vi "WheelTest Dialog Serial with Evt.vi"(8 "error in (no error)":cluster{"状态":bool, "代码":i32, "源":string} caption="错误输入（无错误）", 11 "设置输入":T1) -> (0 "error in (no error) 2":cluster{"状态":bool, "代码":i32, "源":string} caption="错误输入（无错误）", 3 "设置输出":T1)   [LabVIEW 2012, in "Testing.lvlib"]
doc: "使用该模板构建用户界面事件处理设计模式。将模板应用于对话框及其它用户界面。用户也可创建并执行VI可按照与用户界面事件相同方式处理的用户定义事件。"
uses:
  Testing.lvlib
  Settings/Settings.ctl
  Acquisition/Hardware Configuration.ctl
  Acquisition/Signal Type.ctl
  Logging/Logging Configuration.ctl
  User_define/User_define.lvlib
  Acquisition/Acquisition.lvlib
  Logging/Logging.lvlib
  Settings/Settings.lvlib
panel:
  in  "选项卡控件":enum32{"选项卡 1", "选项卡 2"}(tab)
  in  "左后退按钮":bool
  in  "Exit":bool caption="停止"
  in  "左行走轮启停控制":bool caption="按钮1"
  in  "左行走轮速度":u8(slide) scale=0.0..100.0
  out "左行走轮速度反馈值":u16(slide) scale=0.0..100.0
  in  "左前进按钮":bool
  out "右行走轮速度反馈值":u16(slide) scale=0.0..100.0
  in  "右行走轮速度":u8(slide) scale=0.0..100.0
  in  "右行走轮启停控制":bool caption="按钮1"
  in  "右前进按钮":bool
  in  "右后退按钮":bool
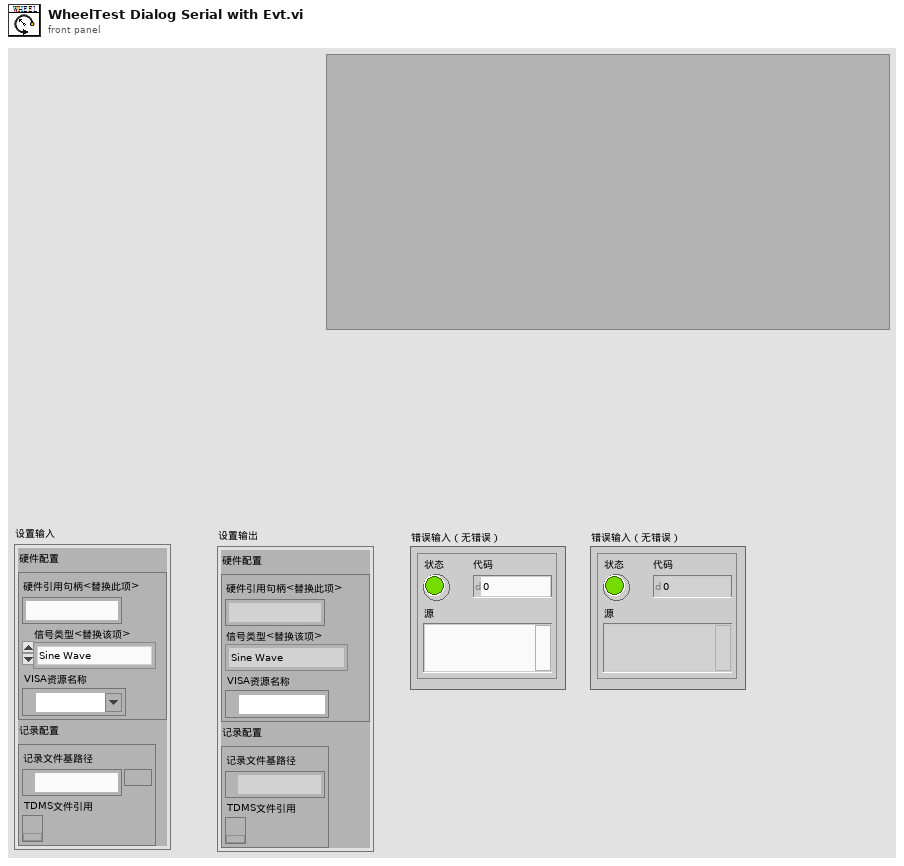
[diagram p1: front panel]
types:
  T1 = typedef "Settings.lvlib/Settings.ctl" = cluster{"硬件配置":T2, "记录配置":T4}
  T2 = typedef "Acquisition.lvlib/Hardware Configuration.ctl" = cluster{"硬件引用句柄<替换此项>":string, "信号类型<替换该项>":T3, "VISA资源名称":refnum<visa-resource-name>}
  T3 = typedef "Acquisition.lvlib/Signal Type.ctl" = enum16{"Sine Wave", "Square with Noise"}
  T4 = typedef "Logging.lvlib/Logging Configuration.ctl" = cluster{"记录文件基路径":path, "TDMS文件引用":refnum<k34>}
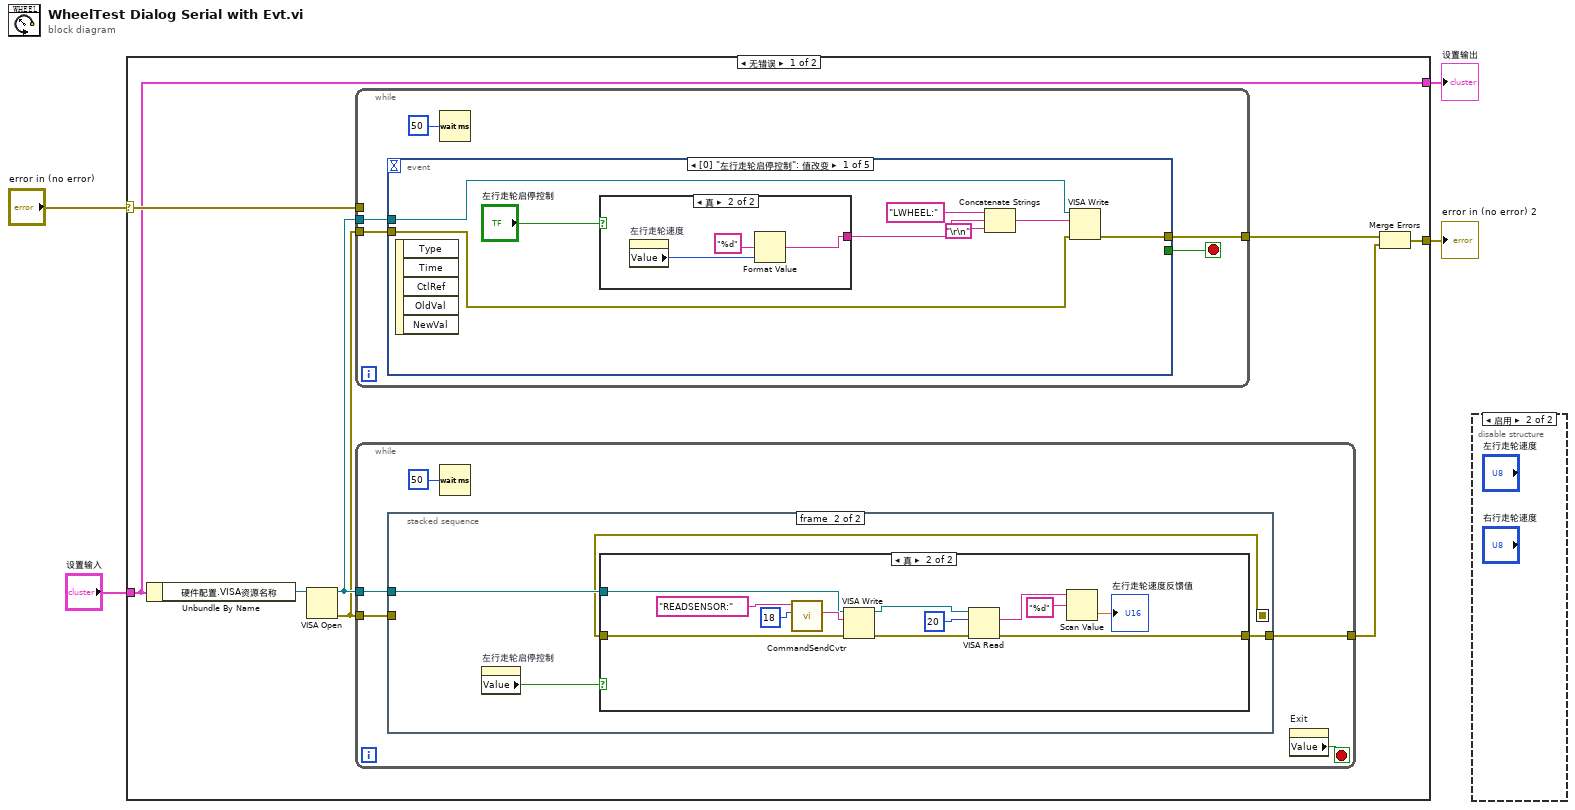
[diagram p0: block diagram]
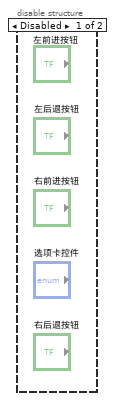
[diagram p2: hidden frame]
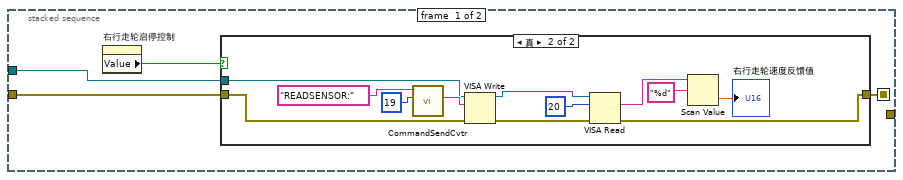
[diagram p3: hidden frame]
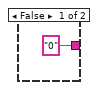
[diagram p6: hidden frame]
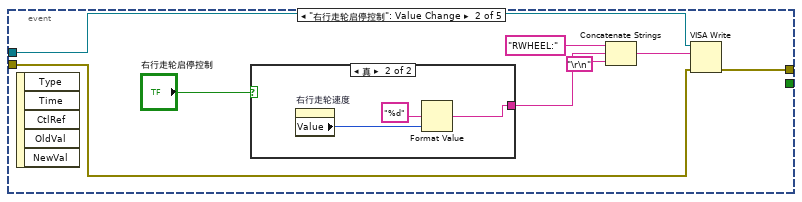
[diagram p7: hidden frame]
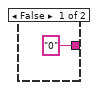
[diagram p8: hidden frame]
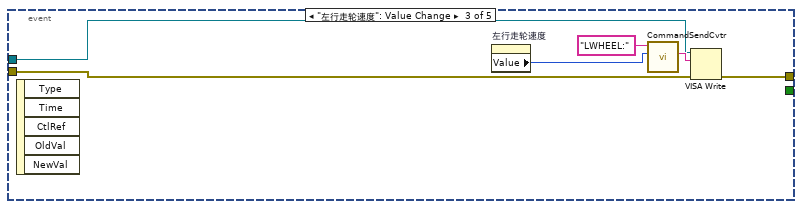
[diagram p9: hidden frame]
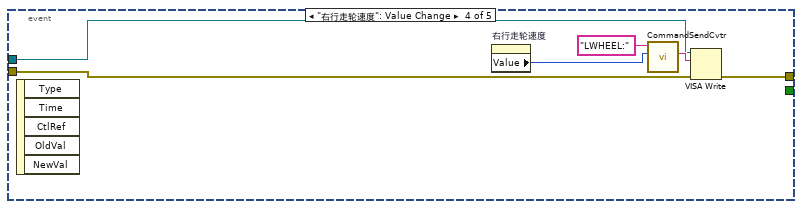
[diagram p10: hidden frame]
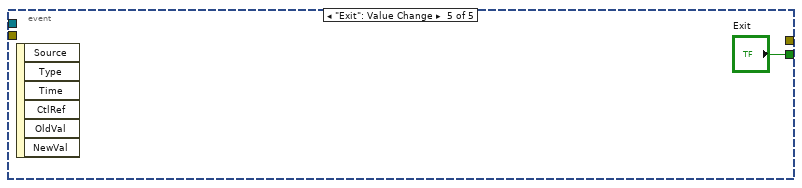
[diagram p11: hidden frame]
diagram:
  n1 = case shown="无错误" "error in (no error)" {
    selector: "error in (no error)" -> [w12 w95]
    tunnel: "设置输入" -> [w5 w94]
    tunnel: [w6 w95] -> w3
    tunnel: [w5 w94] -> w1
    frame No Error {
      n2 = Unbundle By Name(w5) -> ("硬件配置.VISA资源名称"=w11:refnum<visa-resource-name>)
      n3 = VISA Open(VISA resource name=w11) -> (VISA resource name=w10:refnum<visa-resource-name>, error out=w9:errorcluster)  [unwired: 4 in]
      n4 = while {
        tunnel: w12 -> [_]
        tunnel: w10 -> [w54]
        tunnel: w9 -> [w53]
        tunnel: [w52] -> w8
        stop <- w55 stop-if-true
        n5 = event shown="[0] \"左行走轮启停控制\": 值改变" {
          selector: _ -> [_ _ _ _ _]
          dyn-events: _ -> [_ _ _ _ _]
          timeout: _ -> [_ _ _ _ _]
          tunnel: [_ _ _ _ "Exit"] -> w55
          tunnel: [w60 w70 w81 w87 _] -> w52
          tunnel: w54 -> [w59 w72 w83 w89 _]
          tunnel: w53 -> [w58 w71 w82 w88 _]
          event "左行走轮启停控制": Value Change {
            n6 = event-data() -> ()  [unwired: 1 in, 5 out]
            n7 = case shown="真" "左行走轮启停控制" {
              tunnel: ["0" w67] -> w63
              frame False {
              }
              frame True {
                n8 = property on="左行走轮速度" class="Slide (严格)"() -> ("Value"=w66:u8)  [unwired: 2 in, 2 out]
                n9 = Format Value ("格式化值")(format string="%d" ("格式字符串"), value (0)=w66) -> (output string=w67:string)  [unwired: 1 in]
              }
            }
            n10 = Concatenate Strings("LWHEEL:", w63, "\r\n") -> (w61:string)
            n11 = VISA Write(VISA resource name=w59, write buffer=w61, error in (no error)=w58) -> (error out=w60:errorcluster)  [unwired: 2 out]
          }
          event "右行走轮启停控制": Value Change {
            n12 = event-data() -> ()  [unwired: 1 in, 5 out]
            n13 = case shown="真" "右行走轮启停控制" {
              tunnel: ["0" w79] -> w75
              frame False {
              }
              frame True {
                n14 = property on="右行走轮速度" class="Slide (严格)"() -> ("Value"=w78:u8)  [unwired: 2 in, 2 out]
                n15 = Format Value ("格式化值")(format string="%d" ("格式字符串"), value (0)=w78) -> (output string=w79:string)  [unwired: 1 in]
              }
            }
            n16 = Concatenate Strings("RWHEEL:", w75, "\r\n") -> (w73:string)
            n17 = VISA Write(VISA resource name=w72, write buffer=w73, error in (no error)=w71) -> (error out=w70:errorcluster)  [unwired: 2 out]
          }
          event "左行走轮速度": Value Change {
            n18 = event-data() -> ()  [unwired: 1 in, 5 out]
            n19 = property on="左行走轮速度" class="Slide (严格)"() -> ("Value"=w86:u8)  [unwired: 2 in, 2 out]
            n20 = call "CommandSendCvtr.vi"("Para"=w86, "Cmd"="LWHEEL:") -> ("连接的字符串"=w84:string)  [unwired: 9 in]
            n21 = VISA Write(VISA resource name=w83, write buffer=w84, error in (no error)=w82) -> (error out=w81:errorcluster)  [unwired: 2 out]
          }
          event "右行走轮速度": Value Change {
            n22 = event-data() -> ()  [unwired: 1 in, 5 out]
            n23 = property on="右行走轮速度" class="Slide (严格)"() -> ("Value"=w90:u8)  [unwired: 2 in, 2 out]
            n24 = call "CommandSendCvtr.vi"("Para"=w90, "Cmd"="LWHEEL:") -> ("连接的字符串"=w91:string)  [unwired: 9 in]
            n25 = VISA Write(VISA resource name=w89, write buffer=w91, error in (no error)=w88) -> (error out=w87:errorcluster)  [unwired: 2 out]
          }
          event "Exit": Value Change {
            n26 = event-data() -> ()  [unwired: 1 in, 6 out]
          }
        }
        n27 = Wait (ms)(milliseconds to wait=u32 50 ("等待时间（毫秒）")) -> ()  [unwired: 1 out]
      }
      n28 = while {
        tunnel: w10 -> [w16]
        tunnel: w9 -> [w15]
        tunnel: [w14] -> w7
        stop <- w17 stop-if-true
        n29 = stacked-sequence {
          seq-local: [w18 _] -> [_ w36]
          tunnel: w16 -> [w20 w37]
          tunnel: w15 -> [w19 _]
          tunnel: [_ w35] -> w14
          frame #0 {
            n30 = property on="右行走轮启停控制" class="Bool (严格)"() -> ("Value"=w21:bool)  [unwired: 2 in, 2 out]
            n31 = case shown="真" w21 {
              tunnel: w20 -> [_ w25]
              tunnel: w19 -> [w22 w24]
              tunnel: [w22 w23] -> w18
              frame False {
              }
              frame True {
                n32 = call "CommandSendCvtr.vi"("Para"=u8 19, "Cmd"="READSENSOR:") -> ("连接的字符串"=w31:string)  [unwired: 9 in]
                n33 = VISA Write(VISA resource name=w25, write buffer=w31, error in (no error)=w24) -> (VISA resource name out=w34:refnum<visa-resource-name>, error out=w33:errorcluster)  [unwired: 1 out]
                n34 = VISA Read(VISA resource name=w34, byte count=u32 20 ("字节总数"), error in (no error)=w33) -> (read buffer=w28:string, error out=w23:errorcluster)  [unwired: 2 out]
                n35 = Scan Value(string=w28, format string="%d" ("格式字符串")) -> (value=→"右行走轮速度反馈值":dbl)  [unwired: 1 in, 1 out]
              }
            }
          }
          frame #1 {
            n36 = property on="左行走轮启停控制" class="Bool (严格)"() -> ("Value"=w38:bool)  [unwired: 2 in, 2 out]
            n37 = case shown="真" w38 {
              tunnel: [w39 w43] -> w35
              tunnel: w37 -> [_ w42]
              tunnel: w36 -> [w39 w41]
              frame False {
              }
              frame True {
                n38 = call "CommandSendCvtr.vi"("Para"=u8 18, "Cmd"="READSENSOR:") -> ("连接的字符串"=w48:string)  [unwired: 9 in]
                n39 = VISA Write(VISA resource name=w42, write buffer=w48, error in (no error)=w41) -> (VISA resource name out=w51:refnum<visa-resource-name>, error out=w50:errorcluster)  [unwired: 1 out]
                n40 = VISA Read(VISA resource name=w51, byte count=u32 20 ("字节总数"), error in (no error)=w50) -> (read buffer=w45:string, error out=w43:errorcluster)  [unwired: 2 out]
                n41 = Scan Value(string=w45, format string="%d" ("格式字符串")) -> (value=→"左行走轮速度反馈值":dbl)  [unwired: 1 in, 1 out]
              }
            }
          }
        }
        n42 = Wait (ms)(milliseconds to wait=u32 50 ("等待时间（毫秒）")) -> ()  [unwired: 1 out]
        n43 = property on="Exit" class="Bool (严格)"() -> ("Value"=w17:bool)  [unwired: 2 in, 2 out]
      }
      n44 = Merge Errors(w8, w7) -> (w6:errorcluster)
    }
    frame Error {
    }
  }
  "error in (no error) 2" <- w3
  "设置输出" <- w1
  n45 = disable-structure shown="启用" {
    frame Disabled {
    }
    frame Enabled {
    }
  }
